vi "kinectClose.vi"(8 "error in":errorcluster, 11 "KinectSensor References":T1) -> (0 "error out":errorcluster)   [LabVIEW 2014]
uses:
  controls/KinectSensor References.ctl
  Microsoft.Kinect
  C:/Users/iknox/Documents/BodyFrameDataInterface/bin/Debug/BodyFrameDataInterface.dll
  Users/iknox/Documents/BodyFrameDataInterface/bin/Debug/BodyFrameDataInterface.dll
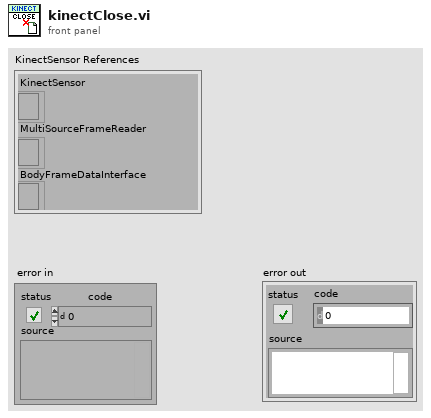
[diagram p1: front panel]
types:
  T1 = typedef "KinectSensor References.ctl" = cluster{"KinectSensor":refnum<k24>, "MultiSourceFrameReader":refnum<k24>, "BodyFrameDataInterface":refnum<k24>}
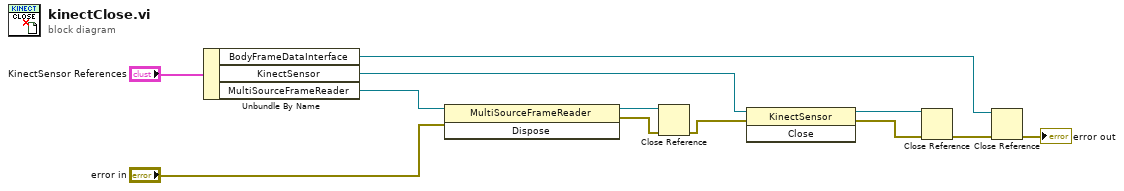
[diagram p0: block diagram]
diagram:
  n1 = Unbundle By Name("KinectSensor References") -> ("BodyFrameDataInterface"=w2:refnum<k24>, "KinectSensor"=w4:refnum<k24>, "MultiSourceFrameReader"=w5:refnum<k24>)
  n2 = invoke class="MultiSourceFrameReader" method="Dispose"(reference=w5, error in="error in") -> (reference out=w12:refnum<k24>, error out=w11:errorcluster)  [unwired: 1 in, 1 out]
  n3 = Close Reference(reference=w12, error in (no error)=w11) -> (error out=w10:errorcluster)
  n4 = invoke class="KinectSensor" method="Close"(reference=w4, error in=w10) -> (reference out=w9:refnum<k24>, error out=w8:errorcluster)  [unwired: 1 in, 1 out]
  n5 = Close Reference(reference=w9, error in (no error)=w8) -> (error out=w3:errorcluster)
  n6 = Close Reference(reference=w2, error in (no error)=w3) -> (error out=→"error out":errorcluster)
